vi "getDescription.vi"(8 "error in (no error)":errorcluster, 11 "Milk in":refnum<class "Milk.lvclass">) -> (0 "error out":errorcluster, 2 "description":string, 3 "Milk out":refnum<class "Milk.lvclass">)   [LabVIEW 2017, in "Milk.lvclass"]
uses:
  Milk.lvclass
  CondimentDecorator/CondimentDecorator.lvclass
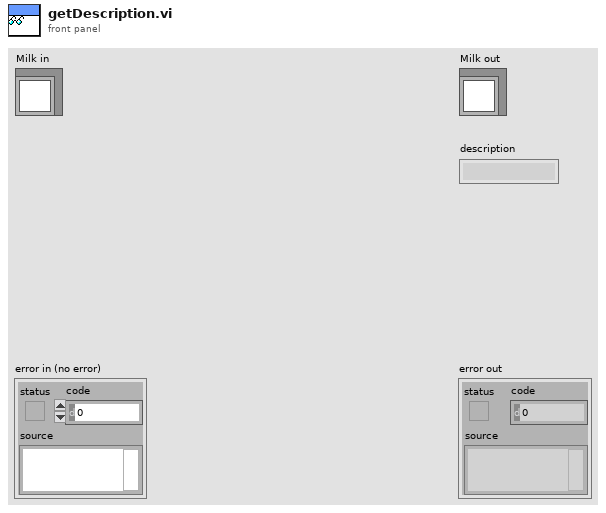
[diagram p1: front panel]
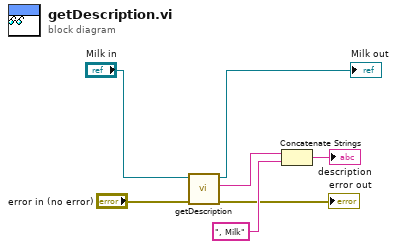
[diagram p0: block diagram]
diagram:
  n1 = call-parent "getDescription.vi"("error in (no error)"="error in (no error)", "CondimentDecorator in"="Milk in") -> ("error out"=→"error out":errorcluster, "description"=w3:string, "CondimentDecorator out"=→"Milk out":refnum<class "Milk.lvclass">)  [unwired: 7 in]
  n2 = Concatenate Strings(w3, ", Milk") -> (→"description":string)
